vi "Start Tracing (Capture to Memory).vi"(8 "error in (no error)":errorcluster) -> (0 "error out":errorcluster)   [LabVIEW 2011, in "NI IO Trace.lvlib"]
doc: "Commands NI I/O Trace to start logging without logging calls to a file. This VI should only be used if a user is going to manually inspect the log on the machine. Otherwise, users should log calls to a file by choosing the Capture to File instance of <B>Start Tracing</B>."
uses:
  <vilib>/NiIOTrace/NI IO Trace.lvlib
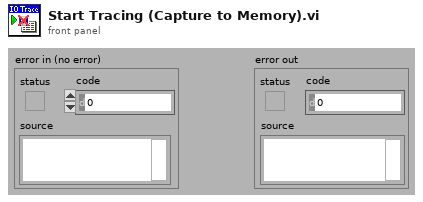
[diagram p1: front panel]
types:
  T1 = enum32{"create", "append or create", "replace or create"}
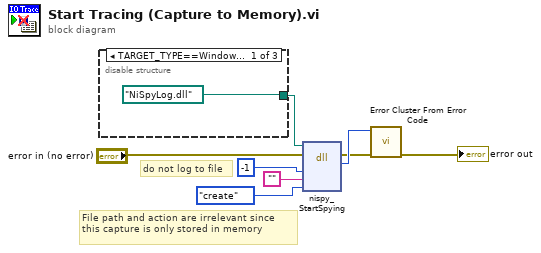
[diagram p0: block diagram]
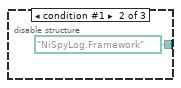
[diagram p2: hidden frame]
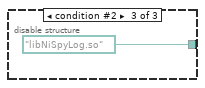
[diagram p3: hidden frame]
diagram:
  # "do not log to file"
  # "File path and action are irrelevant since this capture is only stored in memory"
  n1 = disable-structure shown="TARGET_TYPE==Windows, default" {
    disable-tunnel: [path "NiSpyLog.dll" ("path in") path "NiSpyLog.Framework" ("path in") path "libNiSpyLog.so" ("path in")] -> w6
    frame condition #0 (active) {
    }
    frame condition #1 {
    }
    frame condition #2 {
    }
  }
  n2 = dll-call lib="C:/WINDOWS/system32/NiSpyLog.dll" fn="nispy_StartSpying"(path in=w6, error in="error in (no error)", "logFileSetting"=-1, "filePathString"="", "overwriteFile"=T1."create" ("file write mode (create)")) -> (error out=w5:errorcluster, "return type"=w7:i32)  [unwired: 2 in, 3 out]
  n3 = call <vilib>:"Error Cluster From Error Code.vi"("error in (no error)"=w5, "error code (0)"=w7) -> ("error out"=→"error out":errorcluster)  [unwired: 1 in, 6 out]
